vi "NI9234_simpleUI.vi"() -> ()   [LabVIEW 2020]
uses:
  TYPEDEF/SET_NI9234.ctl
  TYPEDEF/NI9234_TD_MethodSendEventEvent.ctl
  TYPEDEF/NI9234_TD_Method_Queue.ctl
  TYPEDEF/NI9234_TD_MethodNI9234.ctl
  TYPEDEF/NI9234_TD_DataMethod.ctl
panel:
  out "x*y":i32
  out "size(s) 2":i32
  out "size(s)":i32
  in  "SET_NI9234":T1={"IEPE Current value (A)"=0.004, "Sensitivity ACC (mV/g)"=10200.0, "Sample Rate (Sample/sec)"=1000.0, "Samples per Loop"=1000, "file path (use dialog)"=path "", "File Name"="", "Save?"=FALSE} {"Samples per Loop" min=10 max=507900 step=1; "Sample Rate (Sample/sec)" min=400.0 max=51000.0 step=1.0; "Sensitivity ACC (mV/g)" min=5.0 max=500.0; "IEPE Current value (A)" format="%#_13g"}
  out "Waveform Chart":waveform(dbl)[](graph)
  in  "stop":bool
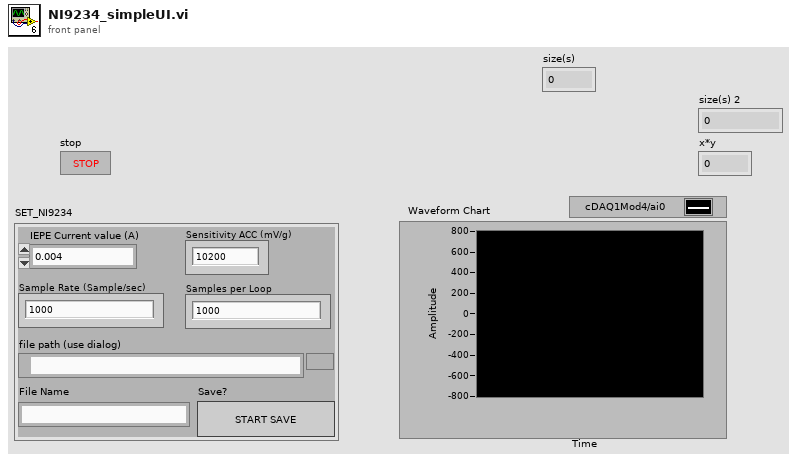
[diagram p1: front panel]
types:
  T1 = typedef "SET_NI9234.ctl" = cluster{"IEPE Current value (A)":dbl, "Sensitivity ACC (mV/g)":dbl, "Sample Rate (Sample/sec)":dbl, "Samples per Loop":i32, "file path (use dialog)":path, "File Name":string, "Save?":bool}
  T2 = typedef "NI9234_TD_DataMethod.ctl" = enum16{"NO_OP", "POPULATE", "USE", "INIT"}
  T3 = typedef "NI9234_TD_MethodNI9234.ctl" = enum16{"NO_OP", "INIT", "SET", "GET", "CLOSE"}
  T4 = typedef "NI9234_TD_Method_Queue.ctl" = enum16{"NO_OP", "CREATE", "POPULATE", "FLUSH", "DESTROY", "DEL_ELEM", "GET_STATUS"}
  T5 = typedef "NI9234_TD_MethodSendEventEvent.ctl" = enum16{"NO_OP", "INIT", "SEND", "CLOSE"}
  T6 = typedef "ClusterSaveData.ctl" = cluster{"VariantValue":variant, "SaveData":T7}
  T7 = typedef "SaveData.ctl" = enum16{"NO_OP", "FUNZIONE", "INVIA_DATI", "RILETTURA"}
  T8 = typedef "MethodEvent.ctl" = enum16{"NO_OP", "EVENTO", "ZERO_POS_REL", "ENABLE_CICLI", "CICLI_ESTENSIONE", "CICLI_RETROAZIONE", "CICLI_Numero", "CICLI_GoToMin", "CICLI_ABORT"}
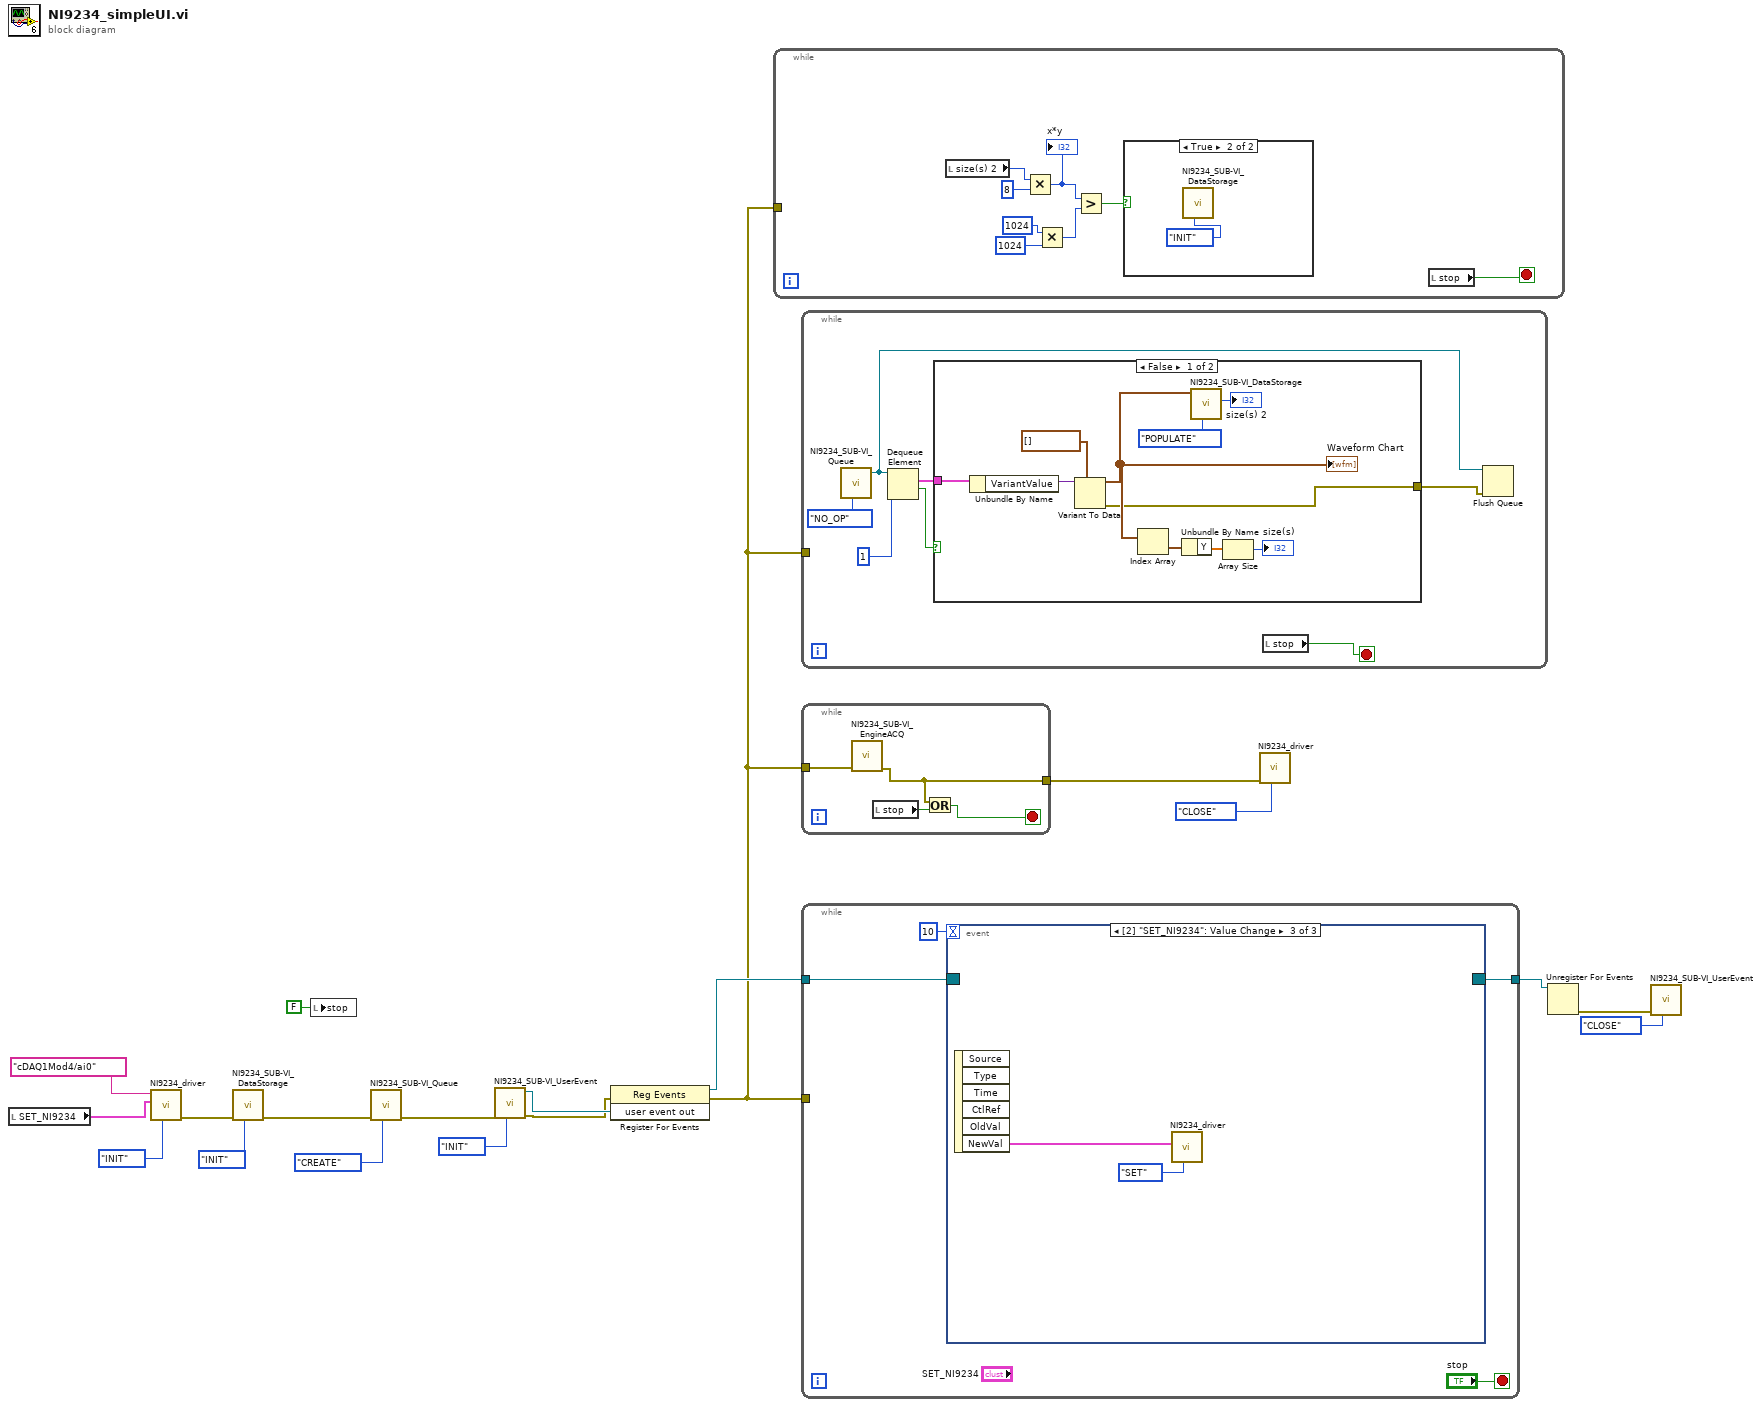
[diagram p0: block diagram]
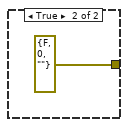
[diagram p3: hidden frame]
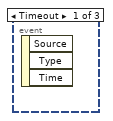
[diagram p4: hidden frame]
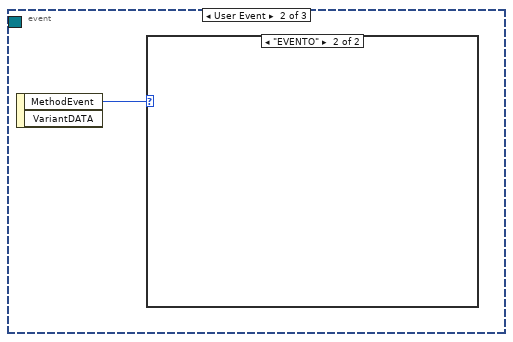
[diagram p5: hidden frame]
diagram:
  n1 = local read "SET_NI9234"() -> (w8:T1)
  n2 = call "NI9234_driver.vi"("Method NI9205"=NI9234_TD_MethodNI9234."INIT", "SET_NI9234"=w8, "Physical Channel"=tag "cDAQ1Mod4/ai0") -> ("error out"=w4:errorcluster)  [unwired: 5 in, 3 out]
  n3 = call "NI9234_SUB-VI_DataStorage.vi"("DataMethod"=NI9234_TD_DataMethod."INIT", "error in (no error)"=w4) -> ("error out"=w3:errorcluster)  [unwired: 7 in, 2 out]
  n4 = local write "stop"(FALSE ("stop")) -> ()
  n5 = call "NI9234_SUB-VI_Queue.vi"("Method"=NI9234_TD_Method_Queue."CREATE", "error in (no error)"=w3) -> ("error out"=w11:errorcluster)  [unwired: 7 in, 2 out]
  n6 = call "NI9234_SUB-VI_UserEvent.vi"("Method_UsE"=NI9234_TD_MethodSendEventEvent."INIT", "error in (no error)"=w11) -> ("error out"=w17:errorcluster, "user event out"=w18:refnum<user-event>)  [unwired: 8 in]
  n7 = register-events(error in=w17, w18) -> (reference out=w19:refnum<event-registration>, error out=w1:errorcluster)  [unwired: 1 in]
  n8 = while {
    tunnel: w1 -> [_]
    stop <- w27 stop-if-true
    n9 = local read "size(s) 2"() -> (w26:i32)
    n10 = Multiply(x=w26, y=8) -> (x*y=w24:i32)
    "x*y" <- w24
    n11 = Multiply(x=1024 ("y"), y=1024) -> (x*y=w21:i32)
    n12 = Greater?(x=w24, y=w21) -> (0:w20:bool)
    n13 = case shown="True" w20 {
      frame False {
      }
      frame True {
        n14 = call "NI9234_SUB-VI_DataStorage.vi"("DataMethod"=NI9234_TD_DataMethod."INIT") -> ()  [unwired: 8 in, 3 out]
      }
    }
    n15 = local read "stop"() -> (w27:bool)
  }
  n16 = while {
    tunnel: w1 -> [_]
    stop <- w31 stop-if-true
    n17 = call "NI9234_SUB-VI_Queue.vi"("Method"=NI9234_TD_Method_Queue."NO_OP") -> ("queue out"=w29:refnum<queue>)  [unwired: 8 in, 2 out]
    n18 = Dequeue Element(queue=w29, timeout in ms (-1)=1) -> (element=w32:T6, timed out?=w33:bool)  [unwired: 1 in, 2 out]
    n19 = case shown="False" w33 {
      tunnel: w32 -> [w45 _]
      tunnel: [w38 errorcluster {"status"=FALSE, "code"=0, "source"=""} ("error out")] -> w30
      frame False {
        n20 = Unbundle By Name(w45) -> ("VariantValue"=w44:variant)
        n21 = Variant To Data(type=waveform(dbl)[] [] ("data"), Variant=w44) -> (data=w39:waveform(dbl)[], error out=w38:errorcluster)  [unwired: 1 in]
        "Waveform Chart" <- w39
        n22 = Index Array(array=w39) -> (element=w42:waveform(dbl))  [unwired: 1 in]
        n23 = Unbundle By Name(w42) -> ("Y"=w41:dbl[])
        n24 = call "NI9234_SUB-VI_DataStorage.vi"("DataMethod"=NI9234_TD_DataMethod."POPULATE", "dataIN"=w39) -> ("size(s)"=→"size(s) 2":i32)  [unwired: 7 in, 2 out]
        n25 = Array Size(array=w41) -> (size(s)=→"size(s)":i32)
      }
      frame True {
      }
    }
    n26 = local read "stop"() -> (w31:bool)
    n27 = Flush Queue(queue=w29, error in (no error)=w30) -> ()  [unwired: 3 out]
  }
  n28 = while {
    tunnel: w1 -> [w50]
    tunnel: [w48] -> w6
    stop <- w47 stop-if-true
    n29 = call "NI9234_SUB-VI_EngineACQ.vi"("error in"=w50) -> ("error out"=w48:errorcluster)  [unwired: 10 in]
    n30 = local read "stop"() -> (w49:bool)
    n31 = Or(x=w48, y=w49) -> (x .or. y?=w47:bool)
  }
  n32 = while {
    tunnel: w19 -> [w54]
    tunnel: w1 -> [_]
    tunnel: [w52] -> w14
    stop <- "stop" stop-if-true
    n33 = event shown="[2] \"SET_NI9234\": Value Change" {
      selector: w54 -> [_ _ _]
      dyn-events: [_ _ _] -> w52
      timeout: 10 -> [_ _ _]
      event Timeout {
        n34 = event-data() -> ()  [unwired: 1 in, 3 out]
      }
      event User Event {
        n35 = event-data() -> ("MethodEvent"=w55:T8)  [unwired: 1 in, 1 out]
        n36 = case shown="\"EVENTO\"" w55 {
          frame "NO_OP", Default {
          }
          frame "EVENTO" {
          }
        }
      }
      event Value Change {
        n37 = event-data() -> ("NewVal"=w56:T1)  [unwired: 1 in, 5 out]
        n38 = call "NI9234_driver.vi"("Method NI9205"=NI9234_TD_MethodNI9234."SET", "SET_NI9234"=w56) -> ()  [unwired: 6 in, 4 out]
      }
    }
  }
  n39 = call "NI9234_driver.vi"("Method NI9205"=NI9234_TD_MethodNI9234."CLOSE", "error in"=w6) -> ()  [unwired: 6 in, 4 out]
  n40 = Unregister For Events(event registration refnum=w14) -> (error out=w13:errorcluster)  [unwired: 1 in]
  n41 = call "NI9234_SUB-VI_UserEvent.vi"("Method_UsE"=NI9234_TD_MethodSendEventEvent."CLOSE", "error in (no error)"=w13) -> ()  [unwired: 8 in, 2 out]
